vi "Read all inputs.vi"(8 "error in (no error)":errorcluster) -> (0 "error out":errorcluster, 2 "inputs":bool[](array[boolean]))   [LabVIEW 2022 SP3]
doc: "Reads input state\n-iologix E1210"
uses:
  <vilib>/NI/Modbus Library/API/Master/Modbus Master.lvclass
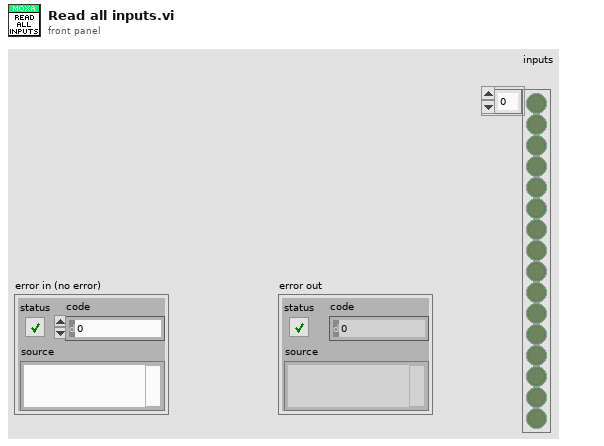
[diagram p1: front panel]
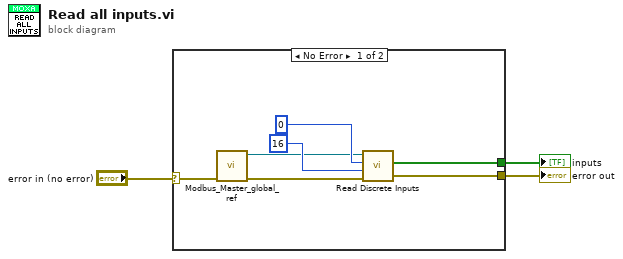
[diagram p0: block diagram]
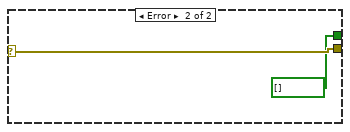
[diagram p2: hidden frame]
diagram:
  n1 = case shown="No Error" "error in (no error)" {
    selector: "error in (no error)" -> [w4 w12]
    tunnel: [w7 bool[] [] ("discrete inputs")] -> w1
    tunnel: [w10 w12] -> w3
    frame No Error {
      n2 = call "Modbus_Master_global_ref.vi"("error in (no error) 2"=w4) -> ("error out 2"=w5:errorcluster, "Modbus Master out"=w6:refnum<class "Modbus Master.lvclass">)  [unwired: 9 in]
      n3 = call-dynamic "Read Discrete Inputs.vi"("error in"=w5, "number of inputs"=u16 16, "starting address"=u16 0, "Modbus master in"=w6) -> ("error out"=w10:errorcluster, "discrete inputs"=w7:bool[])  [unwired: 5 in, 1 out]
    }
    frame Error {
    }
  }
  "error out" <- w3
  "inputs" <- w1
